vi "Banking system.vi"() -> ()   [LabVIEW 2012]
uses:
  Globalvariable.vi
panel:
  out "Account":dbl
  in  "Select Deposit or Withdraw":enum16{"Withdraw", "Deposit"}(ring)
  in  "Enter the Amount":dbl
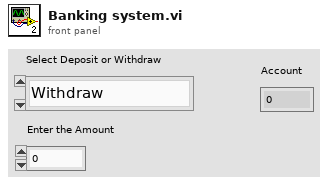
[diagram p1: front panel]
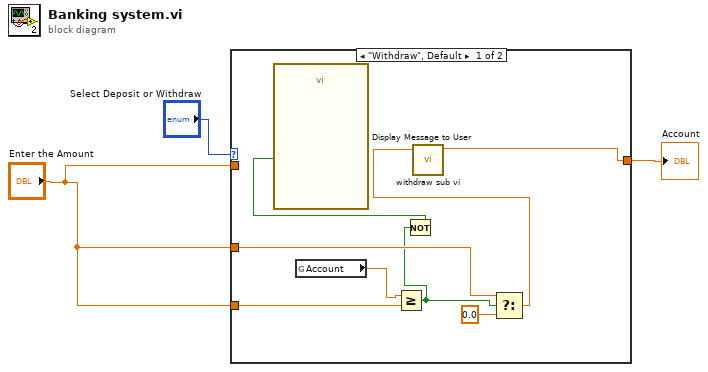
[diagram p0: block diagram]
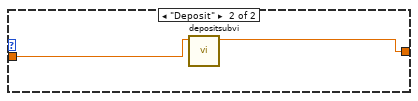
[diagram p2: hidden frame]
diagram:
  n1 = case shown="\"Withdraw\", Default" "Select Deposit or Withdraw" {
    tunnel: [w11 w13] -> w2
    tunnel: "Enter the Amount" -> [_ w12]
    tunnel: "Enter the Amount" -> [w8 _]
    tunnel: "Enter the Amount" -> [w7 _]
    frame "Withdraw", Default {
      n2 = global read "Globalvariable.vi" "Account"() -> (w9:dbl)
      n3 = Greater Or Equal?(x=w9, y=w8) -> (x >= y?=w5:bool)
      n4 = Not(x=w5) -> (.not. x?=w4:bool)
      n5 = call "Display Message to User"("Enable"=w4) -> ()  [unwired: 9 in, 2 out]
      n6 = Select(t=w7, s=w5, f=0.0) -> (s? t:f=w6:dbl)
      n7 = call "withdraw sub vi.vi"("Enter the Amount"=w6) -> ("Numeric"=w11:dbl)  [unwired: 10 in]
    }
    frame "Deposit" {
      n8 = call "depositsubvi.vi"("Enter the Amount"=w12) -> ("Numeric"=w13:dbl)  [unwired: 10 in]
    }
  }
  "Account" <- w2
